vi "Capture.vi"() -> ()   [LabVIEW 2016]
uses:
  <vilib>/rvi/Emulation/niFpgaGetClockAttributes.vi
  <vilib>/rvi/Emulation/niFpgaSctlEmulationGetInTimedLoop.vi
  <vilib>/rvi/Emulation/niFpgaEmulationReportErrorSimple.vi
  <vilib>/rvi/eio/common/nirviEmuTemplateMethod_errors.vi
  <vilib>/rvi/interface/RandomDataEmulation/niFpgaRandomDataHandleErrors.vi
  <vilib>/rvi/Emulation/niFpgaCriticalErrorInLSC.vi
  <vilib>/eio/EIONode/EIONode.xnode
  <vilib>/rvi/DataTransferAndStorage/Container/XNode/niFpgaContainer.xnode
  <vilib>/rvi/interface/RandomDataEmulation/nirviRandomDataFpgaReadWriteTemplate.vi
panel:
  in  "stop":bool
  in  "Count(Ticks)":u32=500000
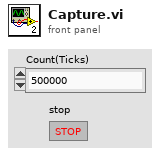
[diagram p1: front panel]
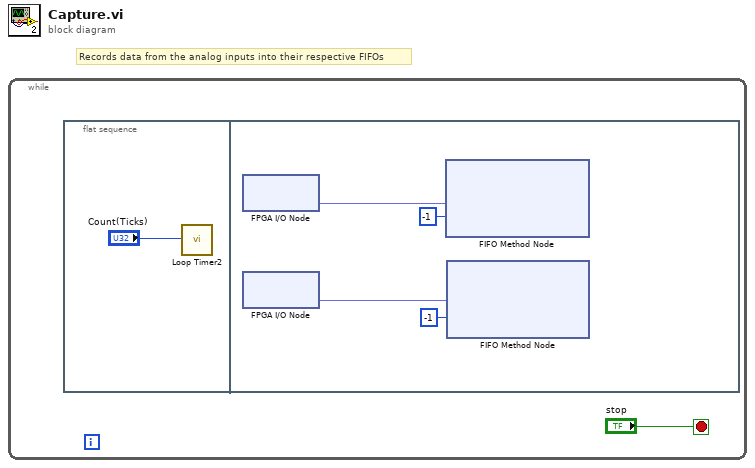
[diagram p0: block diagram]
diagram:
  # "Records data from the analog inputs into their respective FIFOs"
  n1 = while {
    stop <- "stop" stop-if-true
    n2 = flat-sequence {
      frame #0 {
        n3 = call "Loop Timer2"("Count(Ticks)"="Count(Ticks)") -> ()  [unwired: 1 out]
      }
      frame #1 {
        n4 = xnode "FPGA I/O Node"() -> ("AI0"=w6:fxp<+,16,3>)  [unwired: 1 in, 1 out]
        n5 = xnode "FPGA I/O Node"() -> ("AI1"=w5:fxp<+,16,3>)  [unwired: 1 in, 1 out]
        n6 = xnode ("FIFO Method Node")("Element"=w6, "Timeout"=-1) -> ()  [unwired: 1 in, 2 out]
        n7 = xnode ("FIFO Method Node")("Element"=w5, "Timeout"=-1) -> ()  [unwired: 1 in, 2 out]
      }
    }
  }
